vi "Build Tag Name.vi"(8 "error in (no error)":errorcluster, 10 "Resource":string, 11 "Tag":string) -> (0 "error out":errorcluster, 3 "System Tag":string)   [LabVIEW 2017]
uses:
  logger/Logger.lvclass
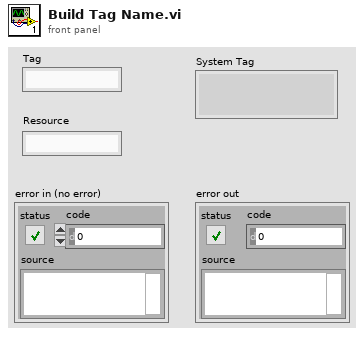
[diagram p1: front panel]
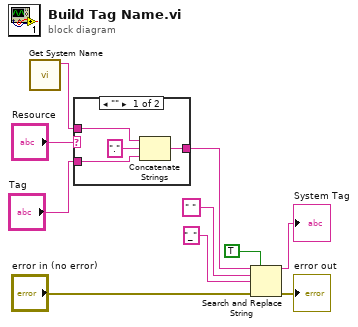
[diagram p0: block diagram]
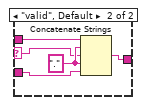
[diagram p2: hidden frame]
diagram:
  n1 = call "Get System Name.vi"() -> ("name"=w4:string)  [unwired: 11 in]
  n2 = case shown="\"\"" "Resource" {
    selector: "Resource" -> [_ w15]
    tunnel: [w11 w19] -> w8
    tunnel: w4 -> [w14 w18]
    tunnel: "Tag" -> [w13 w17]
    frame "" {
      n3 = Concatenate Strings(w14, "." ("element"), w13) -> (w11:string)
    }
    frame "valid", Default {
      w16 = "." ("element")
      n4 = Concatenate Strings(w18, w16, w15, w16, w17) -> (w19:string)
    }
  }
  n5 = Search and Replace String(replace all?=TRUE ("replace all? (F)"), input string=w8, search string=" ", replace string="_" ("replace string (\"\")"), error in="error in (no error)") -> (result string=→"System Tag":string, error out=→"error out":errorcluster)  [unwired: 3 in, 2 out]
